vi "Main VI Path Global.vi"(7 "Write (F)":bool, 8 "Error IN":errorcluster, 11 "Path IN":path) -> (0 "Error OUT":errorcluster, 3 "Path OUT":path)   [LabVIEW 2010]
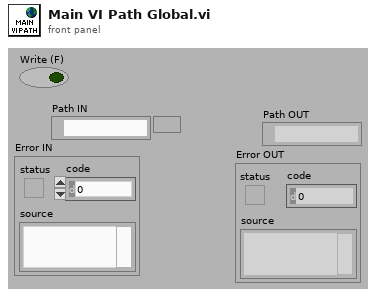
[diagram p1: front panel]
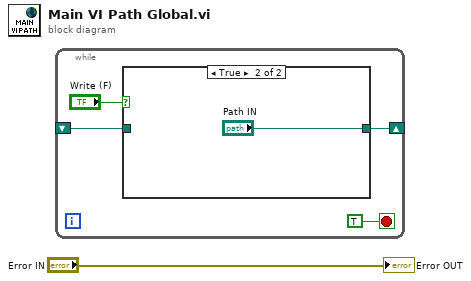
[diagram p0: block diagram]
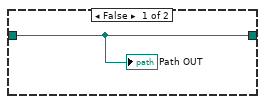
[diagram p2: hidden frame]
diagram:
  n1 = while {
    shift-right: [w3] -> _
    shift-left: _ -> [w2]
    stop <- TRUE stop-if-true
    n2 = case shown="True" "Write (F)" {
      tunnel: [w6 "Path IN"] -> w3
      tunnel: w2 -> [w6 _]
      frame False {
        "Path OUT" <- w6
      }
      frame True {
      }
    }
  }
  "Error OUT" <- "Error IN"
